vi "Get CN Config Enable.vi"(8 "error in (no error)":errorcluster, 9 "Show Tab":refnum<vi>, 10 "CN Pic Ref":refnum<vi>[](array[refnum]), 11 "CN image":T1) -> (0 "error out":errorcluster, 3 "CN image out":T1)   [LabVIEW 2014]
uses:
  Type'def/Tab.ctl
  <vilib>/picture/picture.llb/imagedata.ctl
  Type'def/CN Config Ctr.ctl
  Type'def/CN image Ctr.ctl
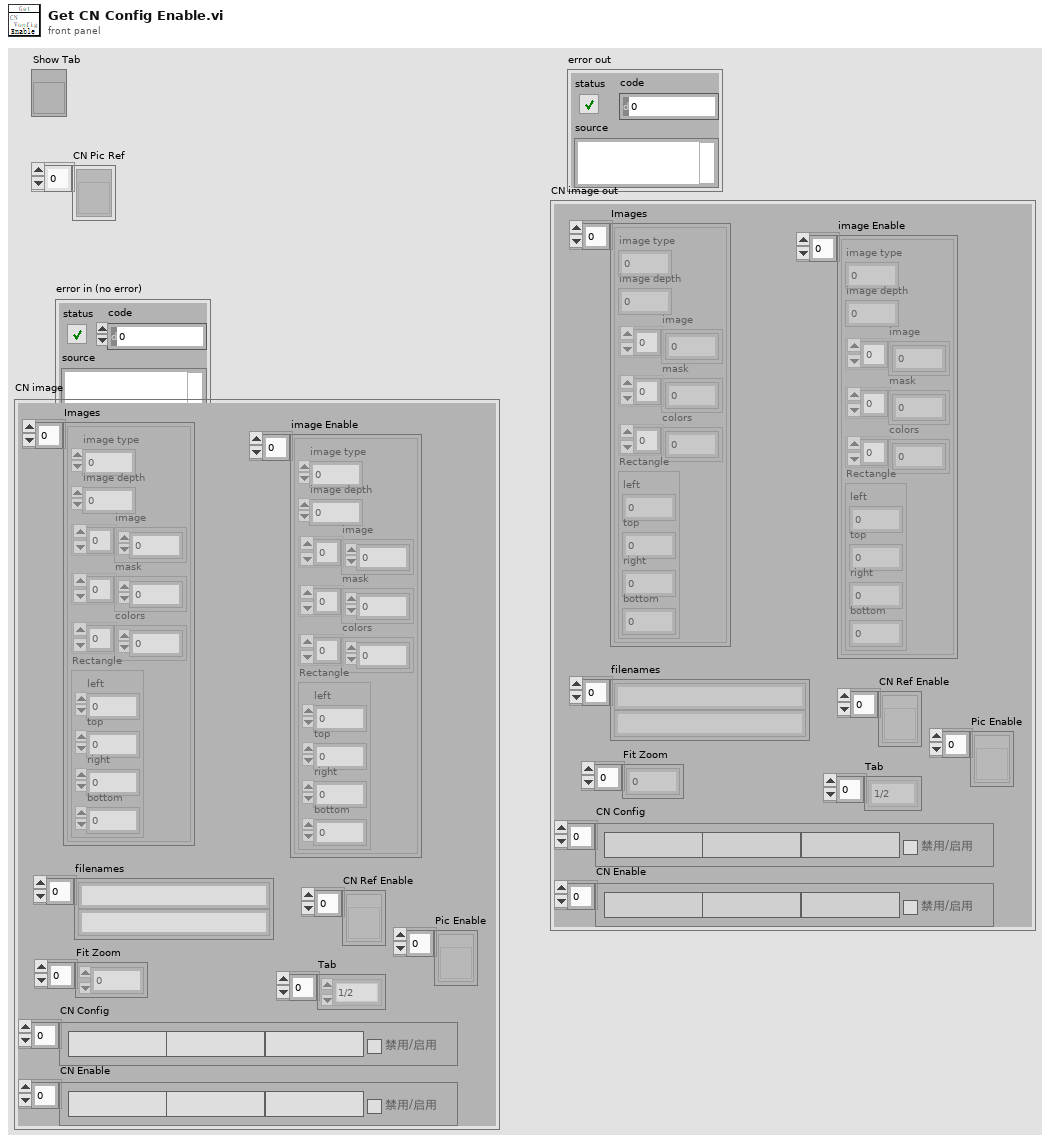
[diagram p1: front panel]
types:
  T1 = typedef "CN image Ctr.ctl" = cluster{"Images":T2[], "filenames":string[], "Fit Zoom":dbl[], "CN Config":T3[], "CN Enable":T3[], "image Enable":T2[], "CN Ref Enable":refnum<vi>[], "Tab ":enum32{"1/2", "1/3", "1/4", "1/5", "2/5", "3/5"}[], "Pic Enable":refnum<vi>[]}
  T2 = typedef "imagedata.ctl" = cluster{"image type":i32, "image depth":i32, "image":u8[], "mask":u8[], "colors":u32[], "Rectangle":cluster{"left":i16, "top":i16, "right":i16, "bottom":i16}}
  T3 = typedef "CN Config Ctr.ctl" = cluster{"Model":string, "Pic_Name":string, "CarName":string, "En/Disable":bool}
  T4 = typedef "Tab.ctl" = enum32{"Customer and Shift Info", "Manufacture Info", "Device error info"}
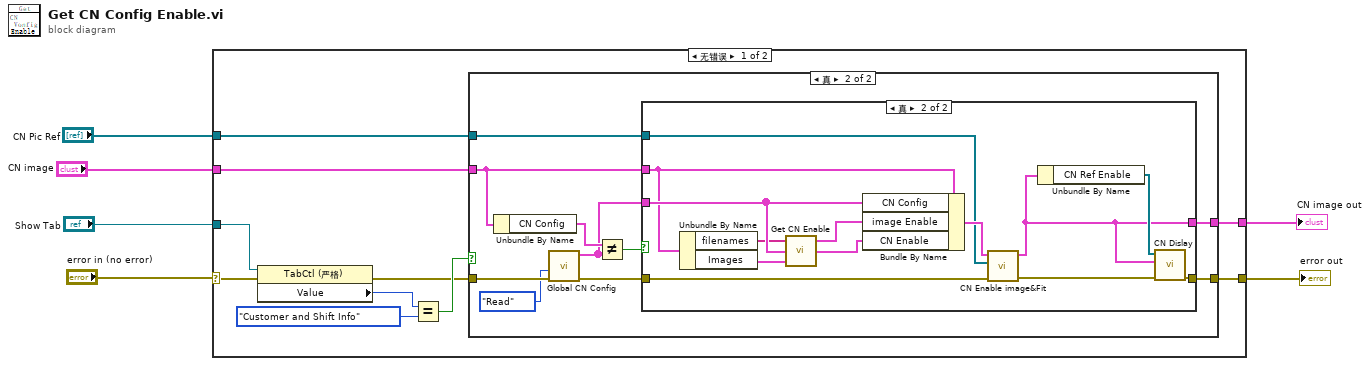
[diagram p0: block diagram]
diagram:
  n1 = case shown="无错误" "error in (no error)" {
    selector: "error in (no error)" -> [w16 w44]
    tunnel: "Show Tab" -> [w15 _]
    tunnel: "CN image" -> [w10 w45]
    tunnel: [w9 w44] -> w3
    tunnel: [w8 w45] -> w2
    tunnel: "CN Pic Ref" -> [w7 _]
    frame No Error {
      n2 = property class="TabCtl (严格)"(reference=w15, error in=w16) -> (error out=w11:errorcluster, "Value"=w13:T4)  [unwired: 1 out]
      n3 = Equal?(x=w13, y=Tab."Customer and Shift Info" ("Value")) -> (x = y?=w12:bool)
      n4 = case shown="真" w12 {
        tunnel: w11 -> [w17 w28]
        tunnel: w10 -> [w18 w25]
        tunnel: [w18 w24] -> w8
        tunnel: [w17 w21] -> w9
        tunnel: w7 -> [_ w22]
        frame False {
        }
        frame True {
          n5 = Unbundle By Name(w25) -> ("CN Config"=w20:T3[])
          n6 = call "Global CN Config.vi"("error in (no error)"=w28, "Mode"=enum16{"Init", "Read", "Write"}."Read") -> ("error out"=w23:errorcluster, "CN Config out"=w19:T3[])  [unwired: 8 in]
          n7 = Not Equal?(x=w20, y=w19) -> (x != y?=w26:bool)
          n8 = case shown="真" w26 {
            tunnel: w25 -> [w30 w42]
            tunnel: w19 -> [_ w43]
            tunnel: [w30 w31] -> w24
            tunnel: w23 -> [w29 w37]
            tunnel: w22 -> [_ w35]
            tunnel: [w29 w34] -> w21
            frame False {
            }
            frame True {
              n9 = Unbundle By Name(w42) -> ("filenames"=w41:string[], "Images"=w40:T2[])
              n10 = call "Get CN Enable.vi"("Images"=w40, "CN Config"=w43, "filenames"=w41) -> ("CN Config out"=w38:T3[], "image Enable"=w39:T2[])  [unwired: 1 in]
              n11 = Bundle By Name(cluster=w42, "CN Config"=w43, "image Enable"=w39, "CN Enable"=w38) -> (w36:T1)
              n12 = call "CN Enable image&Fit.vi"("error in (no error)"=w37, "CN Pic Ref"=w35, "CN image"=w36) -> ("error out"=w33:errorcluster, "CN image out"=w31:T1)  [unwired: 7 in]
              n13 = Unbundle By Name(w31) -> ("CN Ref Enable"=w32:refnum<vi>[])
              n14 = call "CN Dislay.vi"("error in (no error)"=w33, "CN image"=w31, "output array"=w32) -> ("error out"=w34:errorcluster)  [unwired: 8 in]
            }
          }
        }
      }
    }
    frame Error {
    }
  }
  "error out" <- w3
  "CN image out" <- w2
